vi "_db.vi"(7 "command":T1(ring), 8 "error in (no error)":errorcluster, 10 "db in":refnum<k1>, 11 "name":string) -> (0 "error out":errorcluster, 1 "created new?":bool, 3 "db out":refnum<k1>, 4 "info":cluster{"db":refnum<k1>, "Count":i32}, 6 "db list":string[](array[string]))   [LabVIEW 2017, in "TagDB.lvlib"]
doc: "[Covers: REQ_TAGDB_NAMEDDB]"
uses:
  TagDB.lvlib
  Error/_Build Error Cluster.vi
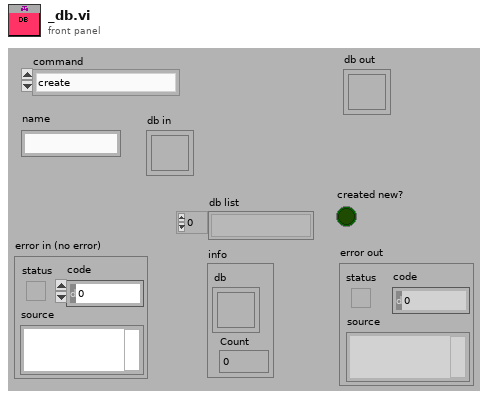
[diagram p1: front panel]
types:
  T1 = enum16{"create", "destroy", "cleanUp", "list", "get info", "force destroy"}
  T2 = typedef "TagDB.lvlib/tagdb-data.ctl" = cluster{"tag-map":variant, "timestamp-map":variant, "namecacher-map":variant, "DataTypeCacher-map":variant, "Tag Adding Lock?":bool, "Global Change Timestamp":timestamp, "Item Change Timestamp":timestamp, "name":string, "Global Change Flag":u64, "Item Change Flag":u64}
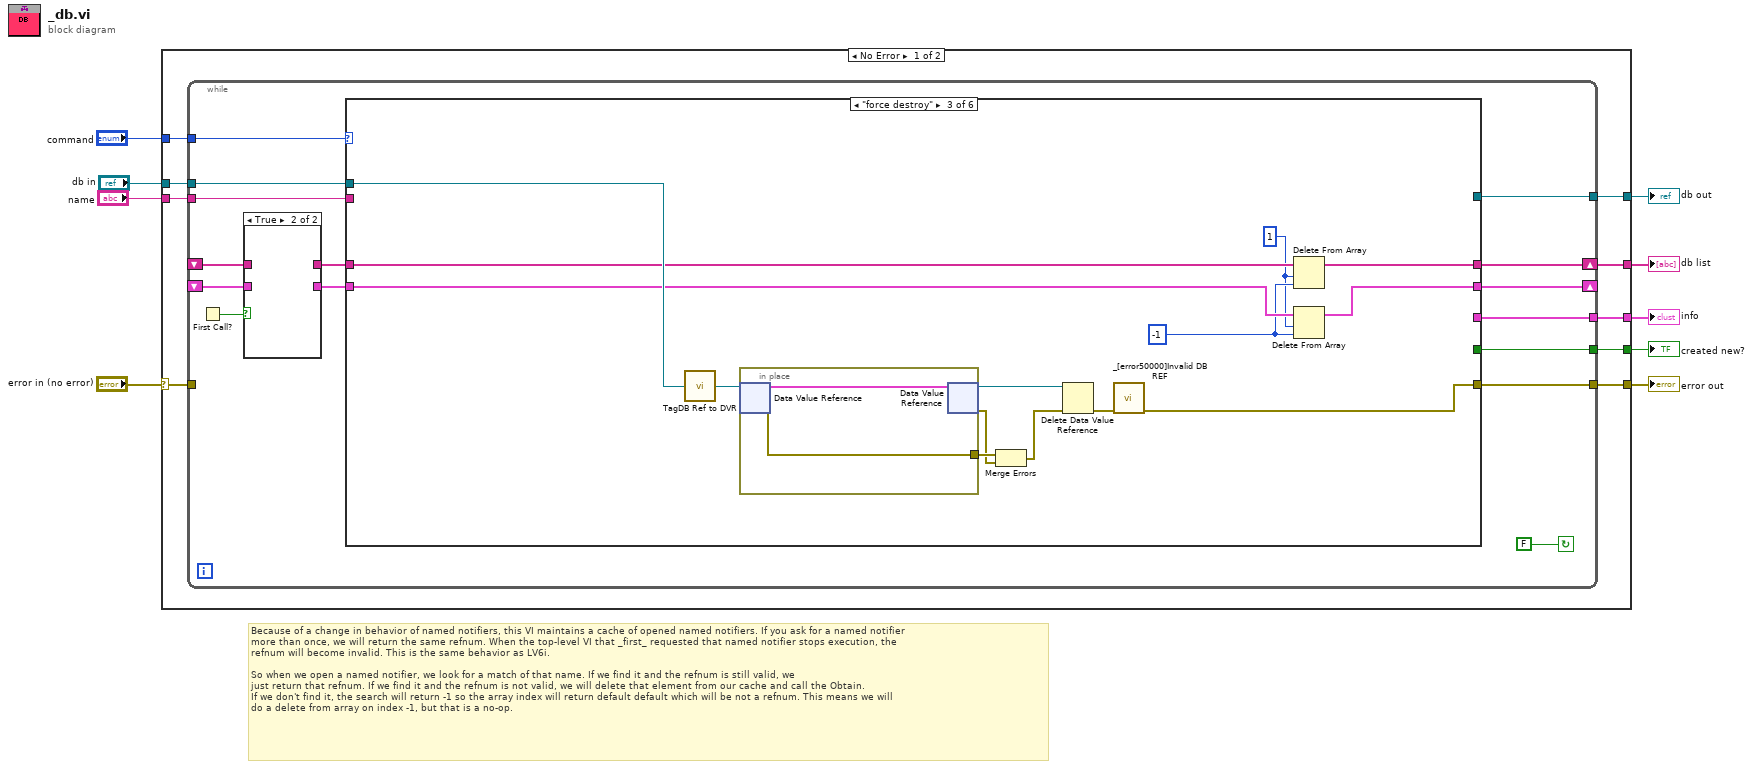
[diagram p0: block diagram]
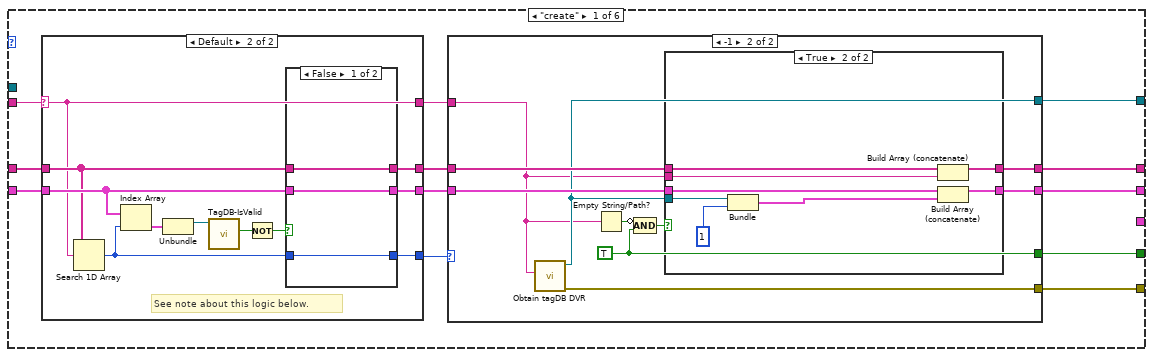
[diagram p3: hidden frame]
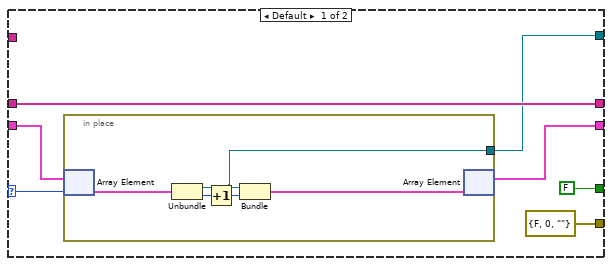
[diagram p4: hidden frame]
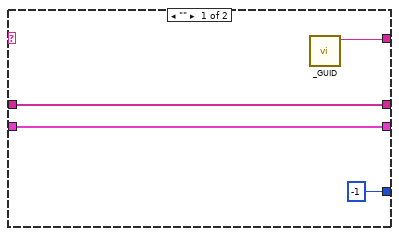
[diagram p6: hidden frame]
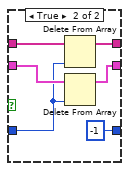
[diagram p7: hidden frame]
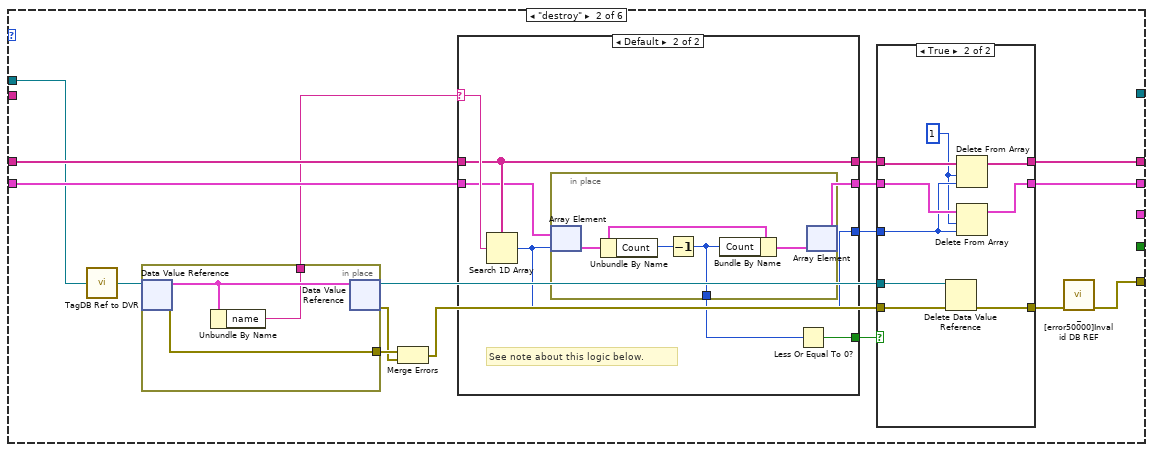
[diagram p8: hidden frame]
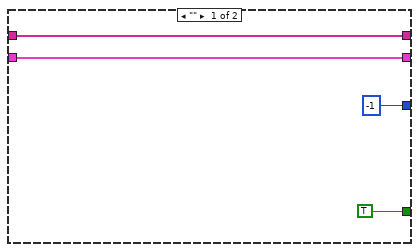
[diagram p10: hidden frame]
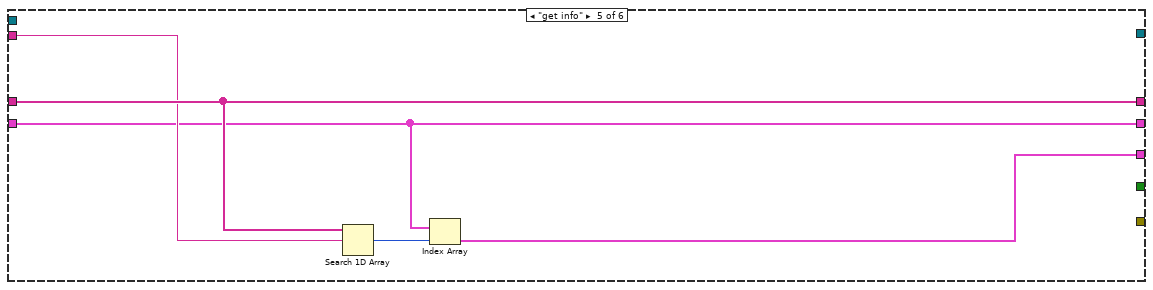
[diagram p12: hidden frame]
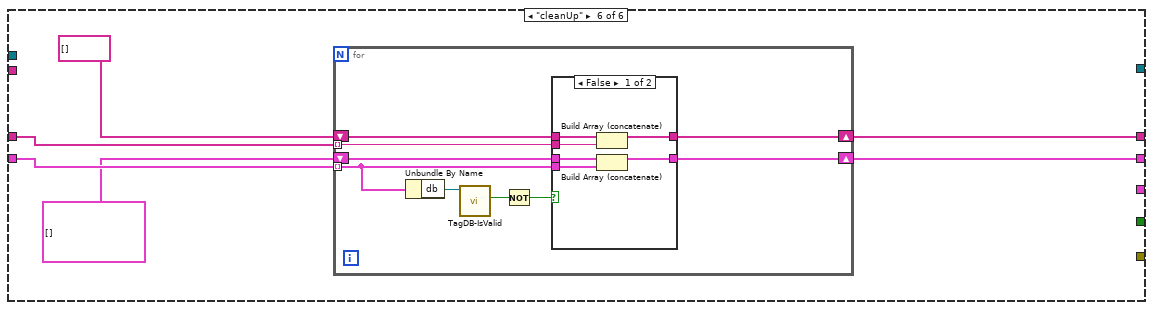
[diagram p13: hidden frame]
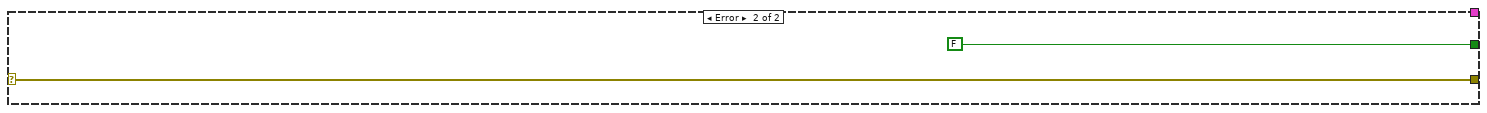
[diagram p15: hidden frame]
diagram:
  # "Because of a change in behavior of named notifiers, this VI maintains a cache of opened named notifiers. If you ask for a named notifier\nmore than once, we will return the same refnum. When the top-level VI that _first_ requested that named notifier stops execution, the\nrefnum will become invalid. This is the same behavior as LV6i.\n\nSo when we open a named notifier, we look for a match of that name. If we find it and the refnum is still valid, we\njust return that refnum. If we find it and the refnum is not valid, we will delete that element from our cache and call the Obtain.\nIf we don't find it, the search will return -1 so the array index will return default default which will be not a refnum. This means we will\ndo a delete from array on index -1, but that is a no-op."
  n1 = case shown="No Error" "error in (no error)" {
    selector: "error in (no error)" -> [w11 w198]
    tunnel: [w18 w198] -> w5
    tunnel: [w17 FALSE ("created new?")] -> w4
    tunnel: [w16 _] -> w9
    tunnel: "name" -> [w15 _]
    tunnel: "command" -> [w14 _]
    tunnel: "db in" -> [w13 _]
    tunnel: [w12 _] -> w2
    tunnel: [w10 _] -> w1
    frame No Error {
      n2 = while {
        shift-right: [w29] -> w12
        shift-left: _ -> [w19]
        shift-right: [w30] -> _
        shift-left: _ -> [w21]
        tunnel: [w33] -> w16
        tunnel: [w32] -> w18
        tunnel: [w31] -> w17
        tunnel: w15 -> [w27]
        tunnel: w14 -> [w24]
        tunnel: w13 -> [w26]
        tunnel: w11 -> [_]
        tunnel: [w25] -> w10
        stop <- FALSE continue-if-true
        n3 = First Call?() -> (First Call?: T/F=w23:bool)
        n4 = case shown="True" w23 {
          tunnel: [w35 _] -> w22
          tunnel: w21 -> [w35 _]
          tunnel: [w34 _] -> w20
          tunnel: w19 -> [w34 _]
          frame False {
          }
          frame True {
          }
        }
        n5 = case shown="\"force destroy\"" w24 {
          tunnel: w20 -> [w46 w120 w155 w168 w173 w176]
          tunnel: w22 -> [w45 w119 w153 w167 w171 w177]
          tunnel: [w44 _ _ _ _ _] -> w33
          tunnel: [w43 w110 w157 _ _ _] -> w32
          tunnel: [w42 _ _ _ _ _] -> w31
          tunnel: [w39 w106 w154 w167 w171 w178] -> w30
          tunnel: [w38 w108 w156 w168 w173 w179] -> w29
          tunnel: w27 -> [w36 _ _ _ w172 _]
          tunnel: w26 -> [_ w115 w161 _ _ _]
          tunnel: [_ _ _ _ w169 _] -> w25
          frame "create" {
            n6 = case shown="Default" w36 {
              selector: w36 -> [_ w88]
              tunnel: [w80 w88] -> w47
              tunnel: w46 -> [w83 w89]
              tunnel: w45 -> [w81 w94]
              tunnel: [w83 w93] -> w37
              tunnel: [w81 w92] -> w40
              tunnel: [-1 ("index") w91] -> w41
              frame "" {
                n7 = call "_GUID.vi"() -> ("uuid"=w80:string)  [unwired: 11 in]
              }
              frame Default {
                # "See note about this logic below."
                n8 = Search 1D Array(1D array=w89, element=w88) -> (index of element=w87:i32)  [unwired: 1 in]
                n9 = Index Array(array=w94, index=w87) -> (element=w86:cluster{"db":refnum<k1>, "Count":i32})
                n10 = Unbundle(w86) -> ("db"=w84:refnum<k1>)  [unwired: 1 out]
                n11 = call "TagDB-IsValid.vi"("TagDB"=w84) -> ("valid TagDB?"=w90:bool)  [unwired: 8 in, 2 out]
                n12 = Not(x=w90) -> (.not. x?=w85:bool)
                n13 = case shown="False" w85 {
                  tunnel: w87 -> [w95 w98]
                  tunnel: w94 -> [w97 w103]
                  tunnel: w89 -> [w96 w102]
                  tunnel: [w96 w101] -> w93
                  tunnel: [w97 w100] -> w92
                  tunnel: [w95 -1 ("index of element")] -> w91
                  frame False {
                  }
                  frame True {
                    n14 = Delete From Array(array=w102, index=w98) -> (array with subset deleted=w101:string[])  [unwired: 1 in, 1 out]
                    n15 = Delete From Array(array=w103, index=w98) -> (array with subset deleted=w100:cluster{"db":refnum<k1>, "Count":i32}[])  [unwired: 1 in, 1 out]
                  }
                }
              }
            }
            n16 = case shown="-1" w41 {
              selector: w41 -> [w49 _]
              tunnel: w47 -> [_ w60]
              tunnel: [w51 w62] -> w44
              tunnel: [errorcluster {"status"=FALSE, "code"=0, "source"=""} ("error out") w69] -> w43
              tunnel: [FALSE ("created new?") w61] -> w42
              tunnel: w40 -> [w50 w65]
              tunnel: [w48 w66] -> w39
              tunnel: [w54 w67] -> w38
              tunnel: w37 -> [w54 w68]
              frame Default {
                n17 = in-place {
                  in-place-border: [w59] -> w51
                  n18 = in-place-array #1(w50, w49) -> (w56:cluster{"db":refnum<k1>, "Count":i32})
                  n19 = Unbundle(w56) -> ("db"=w59:refnum<k1>, "Count"=w58:i32)
                  n20 = Increment(x=w58) -> (x+1=w57:i32)
                  n21 = Bundle("db"=w59, w57) -> (w55:cluster{"db":refnum<k1>, i32})  [unwired: 1 in]
                  n22 = in-place-array #1(w55) -> (w48:cluster{"db":refnum<k1>, "Count":i32}[])  [unwired: 1 out]
                }
              }
              frame -1 {
                w61 = TRUE ("created new?")
                n23 = call "Obtain tagDB DVR.vi"("name"=w60) -> ("error out"=w69:errorcluster, "TagDB"=w62:refnum<k1>)  [unwired: 9 in]
                n24 = Empty String/Path?(string/path=w60) -> (empty?=w64:bool)
                n25 = Compound Arithmetic op=AND(invert w64, w61) -> (w63:bool)
                n26 = case shown="True" w63 {
                  tunnel: w68 -> [w71 w79]
                  tunnel: [w71 w77] -> w67
                  tunnel: [w70 w76] -> w66
                  tunnel: w65 -> [w70 w78]
                  tunnel: w62 -> [_ w73]
                  tunnel: w60 -> [_ w75]
                  frame False {
                  }
                  frame True {
                    n27 = Bundle("TagDB"=w73, 1) -> (w74:cluster{"TagDB":refnum<k1>, i32})  [unwired: 1 in]
                    n28 = Build Array (concatenate)(w79, w75) -> (w77:string[])
                    n29 = Build Array (concatenate)(w78, w74) -> (w76:cluster{"TagDB":refnum<k1>, "Count":i32}[])
                  }
                }
              }
            }
          }
          frame "destroy" {
            n30 = call "TagDB Ref to DVR.vi"("TagDB"=w115) -> ("DVR"=w118:refnum<data-value>)  [unwired: 4 in]
            n31 = in-place {
              in-place-border: [w134] -> w117
              in-place-border: [w133] -> w114
              n32 = in-place-dvr #2(w118) -> (w135:T2, w134:errorcluster)
              n33 = Unbundle By Name(w135) -> ("name"=w133:string)
              n34 = in-place-dvr #2(w135) -> (w112:refnum<data-value>, w116:errorcluster)
            }
            n35 = Merge Errors(w117, w116) -> (w113:errorcluster)
            n36 = case shown="Default" w114 {
              selector: w114 -> [_ w146]
              tunnel: w120 -> [w139 w145]
              tunnel: w119 -> [w138 w141]
              tunnel: [w139 w145] -> w107
              tunnel: [w138 w142] -> w105
              tunnel: [TRUE w144] -> w109
              tunnel: [-1 ("index of element") w140] -> w104
              frame "" {
              }
              frame Default {
                # "See note about this logic below."
                n37 = Search 1D Array(1D array=w145, element=w146) -> (index of element=w140:i32)  [unwired: 1 in]
                n38 = in-place {
                  in-place-border: [w149] -> w143
                  n39 = in-place-array #3(w141, w140) -> (w147:cluster{"db":refnum<k1>, "Count":i32})
                  n40 = Unbundle By Name(w147) -> ("Count"=w150:i32)
                  n41 = Decrement(x=w150) -> (x-1=w149:i32)
                  n42 = Bundle By Name(cluster=w147, "Count"=w149) -> (w148:cluster{"db":refnum<k1>, "Count":i32})
                  n43 = in-place-array #3(w148) -> (w142:cluster{"db":refnum<k1>, "Count":i32}[])  [unwired: 1 out]
                }
                n44 = Less Or Equal To 0?(x=w143) -> (x <= 0?=w144:bool)
              }
            }
            n45 = case shown="True" w109 {
              tunnel: w113 -> [w123 w132]
              tunnel: w112 -> [_ w131]
              tunnel: [w123 w130] -> w111
              tunnel: [w122 w128] -> w108
              tunnel: w107 -> [w122 w129]
              tunnel: [w121 w126] -> w106
              tunnel: w105 -> [w121 w127]
              tunnel: w104 -> [_ w125]
              frame False {
              }
              frame True {
                w124 = 1 ("length")
                n46 = Delete Data Value Reference(data value reference=w131, error in=w132) -> (error out=w130:errorcluster)  [unwired: 1 out]
                n47 = Delete From Array(array=w129, length=w124, index=w125) -> (array with subset deleted=w128:string[])  [unwired: 1 out]
                n48 = Delete From Array(array=w127, length=w124, index=w125) -> (array with subset deleted=w126:cluster{"db":refnum<k1>, "Count":i32}[])  [unwired: 1 out]
              }
            }
            n49 = call "_[error50000]Invalid DB REF.vi"("error in (no error)"=w111) -> ("error out"=w110:errorcluster)  [unwired: 10 in]
          }
          frame "force destroy" {
            w151 = 1 ("length")
            w152 = -1 ("index of element")
            n50 = call "TagDB Ref to DVR.vi"("TagDB"=w161) -> ("DVR"=w164:refnum<data-value>)  [unwired: 4 in]
            n51 = in-place {
              in-place-border: [w165] -> w163
              n52 = in-place-dvr #4(w164) -> (w166:T2, w165:errorcluster)
              n53 = in-place-dvr #4(w166) -> (w159:refnum<data-value>, w162:errorcluster)
            }
            n54 = Merge Errors(w163, w162) -> (w160:errorcluster)
            n55 = Delete Data Value Reference(data value reference=w159, error in=w160) -> (error out=w158:errorcluster)  [unwired: 1 out]
            n56 = call "_[error50000]Invalid DB REF.vi"("error in (no error)"=w158) -> ("error out"=w157:errorcluster)  [unwired: 10 in]
            n57 = Delete From Array(array=w155, length=w151, index=w152) -> (array with subset deleted=w156:string[])  [unwired: 1 out]
            n58 = Delete From Array(array=w153, length=w151, index=w152) -> (array with subset deleted=w154:cluster{"db":refnum<k1>, "Count":i32}[])  [unwired: 1 out]
          }
          frame "list" {
          }
          frame "get info" {
            n59 = Search 1D Array(1D array=w173, element=w172) -> (index of element=w170:i32)  [unwired: 1 in]
            n60 = Index Array(array=w171, index=w170) -> (element=w169:cluster{"db":refnum<k1>, "Count":i32})
          }
          frame "cleanUp" {
            n61 = for {
              shift-right: [w187] -> w179
              shift-left: string[] [] -> [w188]
              tunnel: w177 -> [w182] mode=indexing
              shift-right: [w186] -> w178
              shift-left: cluster{"db":refnum<k1>, "Count":i32}[] [] -> [w184]
              tunnel: w176 -> [w185] mode=indexing
              n62 = Unbundle By Name(w182) -> ("db"=w180:refnum<k1>)
              n63 = call "TagDB-IsValid.vi"("TagDB"=w180) -> ("valid TagDB?"=w183:bool)  [unwired: 8 in, 2 out]
              n64 = Not(x=w183) -> (.not. x?=w181:bool)
              n65 = case shown="False" w181 {
                tunnel: w188 -> [w194 w196]
                tunnel: w182 -> [w190 _]
                tunnel: [w193 w196] -> w187
                tunnel: [w191 w195] -> w186
                tunnel: w185 -> [w192 _]
                tunnel: w184 -> [w189 w195]
                frame False {
                  n66 = Build Array (concatenate)(w194, w192) -> (w193:string[])
                  n67 = Build Array (concatenate)(w189, w190) -> (w191:cluster{"db":refnum<k1>, "Count":i32}[])
                }
                frame True {
                }
              }
            }
          }
        }
      }
    }
    frame Error {
    }
  }
  "created new?" <- w4
  "error out" <- w5
  "db out" <- w9
  "db list" <- w2
  "info" <- w1
